vi "FIO_parse line.vi"(11 "lines":string[](array[string])) -> (1 "stats":cluster{i32, T1}[](array[cluster]), 2 "sum-up":cluster{timestamp, T1}[](array[cluster]) {"?" format="%<%Hh%Mm%S%3u>T"}, 3 "full story":cluster{timestamp, T1}[](array[cluster]) {"?" format="%<%Hh%Mm%S%3u>T"})   [LabVIEW 2014]
uses:
  Controls/TDE_Type.ctl
  Controls/TDE_Type_2.ctl
  Applications/National Instruments/LabVIEW 2015 64-bit/user.lib/_OpenG.lib/array/array.llb/Filter 1D Array with Scalar (I32)__ogtk.vi
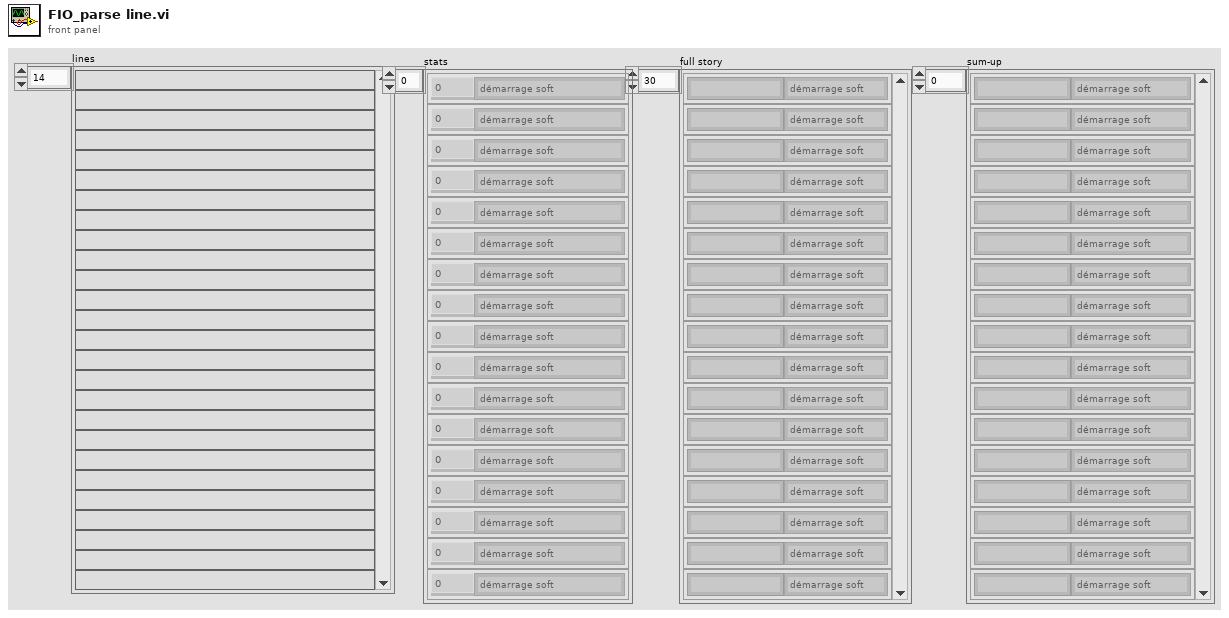
[diagram p1: front panel]
types:
  T1 = typedef "TDE_Type_2.ctl" = enum8{"démarrage soft", "start prod", "Mire", "start cames", "stop cames", "RàZ Vision", "en marche", "P2 ok", "acqFail embout", "acqFail profil", "acqFail collerette", "error open", "error get image", "error 2", "error 3", "error 4", "error 5", "autre"}
  T2 = typedef "TDE_Type.ctl" = enum16{"info", "error", "Mire"}
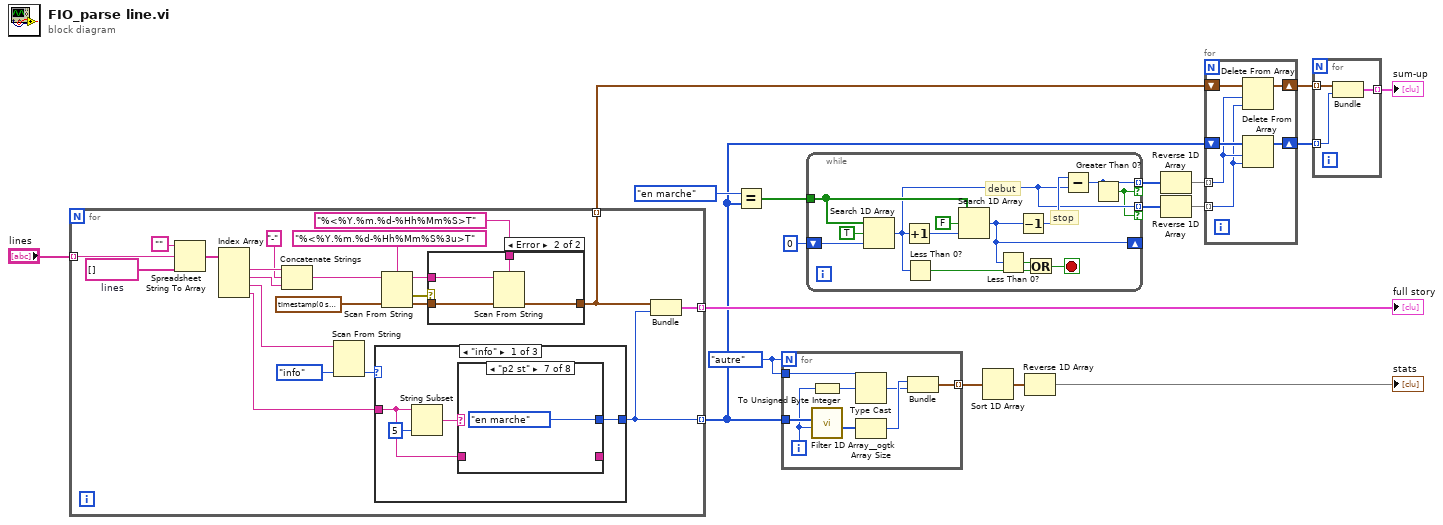
[diagram p0: block diagram]
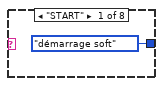
[diagram p3: hidden frame]
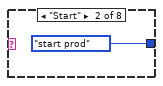
[diagram p4: hidden frame]
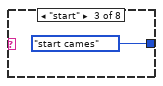
[diagram p5: hidden frame]
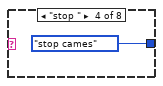
[diagram p6: hidden frame]
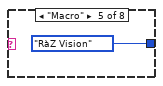
[diagram p7: hidden frame]
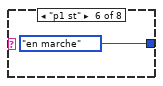
[diagram p8: hidden frame]
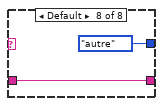
[diagram p9: hidden frame]
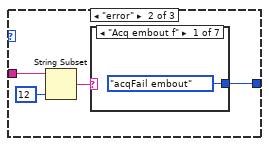
[diagram p10: hidden frame]
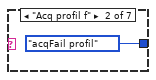
[diagram p11: hidden frame]
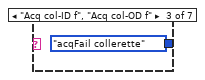
[diagram p12: hidden frame]
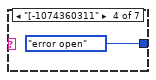
[diagram p13: hidden frame]
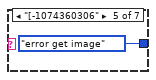
[diagram p14: hidden frame]
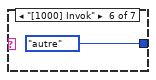
[diagram p15: hidden frame]
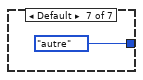
[diagram p16: hidden frame]
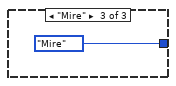
[diagram p17: hidden frame]
diagram:
  w17 = TDE_Type_2."autre"
  n1 = for {
    tunnel: "lines" -> [w38] mode=indexing
    tunnel: [w25] -> w9 mode=indexing
    tunnel: [w24] -> w13 mode=indexing
    tunnel: [w22] -> w6 mode=indexing
    w37 = string[] []  # lines
    n2 = Spreadsheet String To Array(format string="", spreadsheet string=w38, array type (2D Dbl)=w37) -> (array=w33:string[])  [unwired: 1 in]
    n3 = Index Array(array=w33) -> (element #1=w32:string, element #2=w31:string, element #3=w29:string, element #4=w27:string)  [unwired: 4 in]
    n4 = Concatenate Strings(w32, "-", w31) -> (w20:string)
    n5 = Scan From String(input string=w29, default 1=TDE_Type."info") -> (output 1=w26:T2)  [unwired: 3 in, 3 out]
    n6 = case shown="\"info\"" w26 {
      tunnel: w27 -> [w44 w57 _]
      tunnel: [w45 w58 TDE_Type_2."Mire"] -> w25
      frame "info" {
        n7 = String Subset(string=w44, length (rest)=5 ("length (rest)")) -> (substring=w46:string)  [unwired: 1 in]
        n8 = case shown="\"p2 st\"" w46 {
          tunnel: [TDE_Type_2."démarrage soft" TDE_Type_2."start prod" TDE_Type_2."start cames" TDE_Type_2."stop cames" TDE_Type_2."RàZ Vision" TDE_Type_2."en marche" TDE_Type_2."en marche" TDE_Type_2."autre"] -> w45
          tunnel: [_ _ _ _ _ _ _ w55] -> _
          tunnel: w44 -> [_ _ _ _ _ _ _ w55]
          frame "START" {
          }
          frame "Start" {
          }
          frame "start" {
          }
          frame "stop " {
          }
          frame "Macro" {
          }
          frame "p1 st" {
          }
          frame "p2 st" {
          }
          frame Default {
          }
        }
      }
      frame "error" {
        n9 = String Subset(string=w57, length (rest)=12 ("length (rest)")) -> (substring=w59:string)  [unwired: 1 in]
        n10 = case shown="\"Acq embout f\"" w59 {
          tunnel: [TDE_Type_2."acqFail embout" TDE_Type_2."acqFail profil" TDE_Type_2."acqFail collerette" TDE_Type_2."error open" TDE_Type_2."error get image" TDE_Type_2."autre" TDE_Type_2."autre"] -> w58
          frame "Acq embout f" {
          }
          frame "Acq profil f" {
          }
          frame "Acq col-ID f", "Acq col-OD f" {
          }
          frame "[-1074360311" {
          }
          frame "[-1074360306" {
          }
          frame "[1000] Invok" {
          }
          frame Default {
          }
        }
      }
      frame "Mire" {
      }
    }
    n11 = Scan From String(format string="%<%Y.%m.%d-%Hh%Mm%S%3u>T", input string=w20, default 1=timestamp(0 s since 1904-01-01)) -> (error out=w21:errorcluster, output 1=w23:timestamp)  [unwired: 2 in, 2 out]
    n12 = case shown="Error" w21 {
      tunnel: w23 -> [w39 w43]
      tunnel: [w39 w41] -> w22
      tunnel: w20 -> [_ w42]
      tunnel: "%<%Y.%m.%d-%Hh%Mm%S>T" ("format string") -> [_ w40]
      frame No Error {
      }
      frame Error {
        n13 = Scan From String(format string=w40, input string=w42, default 1=w43) -> (output 1=w41:timestamp)  [unwired: 2 in, 3 out]
      }
    }
    n14 = Bundle(w22, w25) -> (w24:cluster{timestamp, T1})  [unwired: 1 in]
  }
  "full story" <- w13
  n15 = Equal?(x=TDE_Type_2."en marche" ("element"), y=w9) -> (x = y?=w10:bool[])
  n16 = for {
    N: w17 -> [_]
    tunnel: w9 -> [w76]
    tunnel: w17 -> [w73]
    tunnel: [w69] -> w16 mode=indexing
    i -> [w74]
    n17 = To Unsigned Byte Integer(number=w74) -> (unsigned 8bit integer=w72:u8)
    n18 = call-poly "Filter 1D Array__ogtk.vi"("items to filter"=w74, "array"=w76) -> ("filtered item indices"=w75:i32[])  [unwired: 4 in, 1 out]
    n19 = Type Cast(type=w73, x=w72) -> (*(type *) &x=w70:T1)
    n20 = Array Size(array=w75) -> (size(s)=w71:i32)
    n21 = Bundle(w71, w70) -> (w69:cluster{i32, T1})  [unwired: 1 in]
  }
  n22 = while {
    tunnel: w10 -> [w89]
    shift-right: [w79] -> _
    shift-left: 0 ("index of element") -> [w88]
    tunnel: [w80] -> w8 mode=indexing if=w77
    tunnel: [w78] -> w7 mode=indexing if=w77
    stop <- w82 stop-if-true
    # "stop"
    # "debut"
    n23 = Search 1D Array(1D array=w89, element=TRUE, start index (0)=w88) -> (index of element=w78:i32)
    n24 = Increment(x=w78) -> (x+1=w85:i32)
    n25 = Less Than 0?(x=w78) -> (x < 0?=w83:bool)
    n26 = Search 1D Array(1D array=w89, element=FALSE, start index (0)=w85) -> (index of element=w79:i32)
    n27 = Less Than 0?(x=w79) -> (x < 0?=w84:bool)
    n28 = Decrement(x=w79) -> (x-1=w81:i32)
    n29 = Or(x=w84, y=w83) -> (x .or. y?=w82:bool)
    n30 = Subtract(x=w81, y=w78) -> (x-y=w80:i32)
    n31 = Greater Than 0?(x=w80) -> (x > 0?=w77:bool)
  }
  n32 = Sort 1D Array(array=w16) -> (sorted array=w15:cluster{i32, T1}[])
  n33 = Reverse 1D Array(array=w15) -> (reversed array=→"stats":cluster{i32, T1}[])
  n34 = Reverse 1D Array(array=w8) -> (reversed array=w2:i32[])
  n35 = Reverse 1D Array(array=w7) -> (reversed array=w1:i32[])
  n36 = for {
    tunnel: w2 -> [w91] mode=indexing
    shift-right: [w94] -> w4
    shift-left: w9 -> [w95]
    tunnel: w1 -> [w90] mode=indexing
    shift-right: [w92] -> w5
    shift-left: w6 -> [w93]
    n37 = Delete From Array(array=w93, length=w91, index=w90) -> (array with subset deleted=w92:timestamp[])  [unwired: 1 out]
    n38 = Delete From Array(array=w95, length=w91, index=w90) -> (array with subset deleted=w94:T1[])  [unwired: 1 out]
  }
  n39 = for {
    tunnel: w5 -> [w98] mode=indexing
    tunnel: w4 -> [w97] mode=indexing
    tunnel: [w96] -> w3 mode=indexing
    n40 = Bundle(w98, w97) -> (w96:cluster{timestamp, T1})  [unwired: 1 in]
  }
  "sum-up" <- w3
